vi "testvi.vi"() -> ()   [LabVIEW 2024]
panel:
  in  "stop":bool
  out "Read":T1
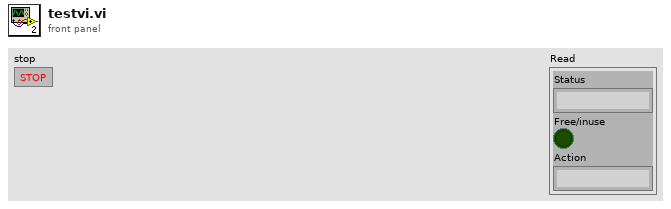
[diagram p1: front panel]
types:
  T1 = cluster{"Status":string, "Free/inuse":bool, "Action":string}
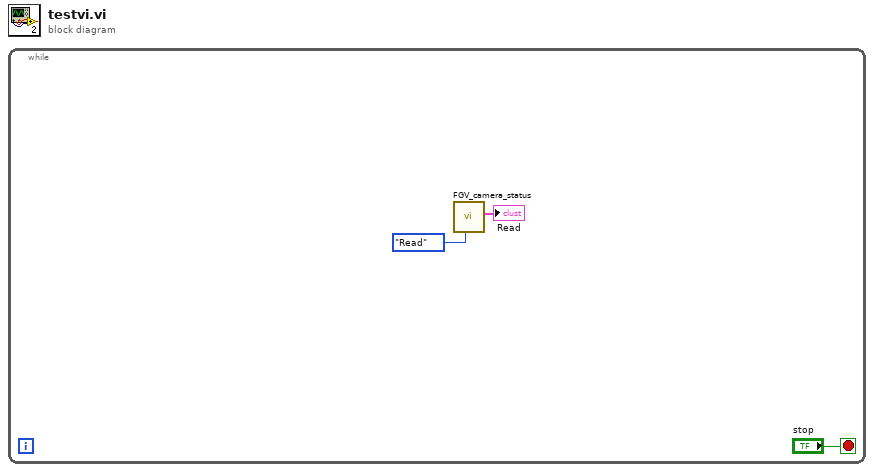
[diagram p0: block diagram]
diagram:
  n1 = while {
    stop <- "stop" stop-if-true
    n2 = call "FGV_camera_status.vi"("Enum"=enum16{"Init", "Read", "Write"}."Read") -> ("Read"=→"Read":T1)  [unwired: 10 in]
  }
